vi "Cut Strings.vi"(8 "error in (no error)":errorcluster, 9 "To Cut":string, 11 "Input String":string) -> (0 "error out":errorcluster, 3 "Output String":string)   [LabVIEW 2018, in "Data Operations.lvlib"]
uses:
  Data Operations.lvlib
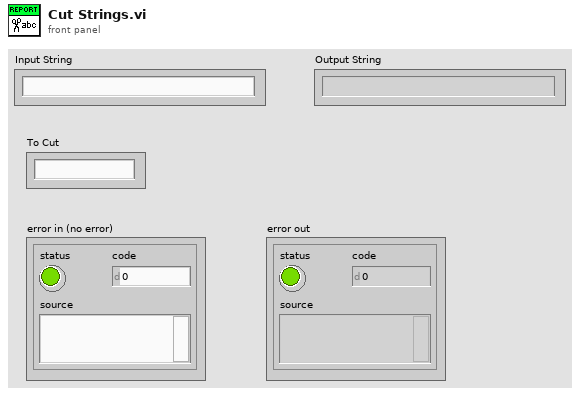
[diagram p1: front panel]
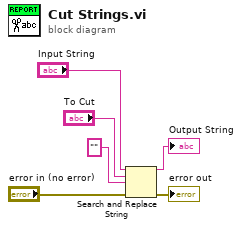
[diagram p0: block diagram]
diagram:
  n1 = Search and Replace String(input string="Input String", search string="To Cut", replace string="" ("replace string (\"\")"), error in="error in (no error)") -> (result string=→"Output String":string, error out=→"error out":errorcluster)  [unwired: 4 in, 2 out]
